vi "CreateCustomScale.vi"(8 "error in (no error)":errorcluster, 11 "DAQmx-AI":refnum<class "DAQmx-AI.lvclass">) -> (0 "error out":errorcluster, 1 "Custom Scaling":bool, 2 "Custom Scale":tag, 3 "DAQmx-AI out":refnum<class "DAQmx-AI.lvclass">)   [LabVIEW 2016, in "DAQmx-AI.lvclass"]
uses:
  DAQmx-AI.lvclass
  <vilib>/DAQmx/create/scale.llb/DAQmx Create Scale (Map Ranges).vi
  <vilib>/DAQmx/create/scale.llb/DAQmx Create Scale (Linear).vi
  <vilib>/DAQmx/create/scale.llb/DAQmx Create Scale (Polynomial).vi
  <vilib>/DAQmx/create/scale.llb/DAQmx Create Scale (Table).vi
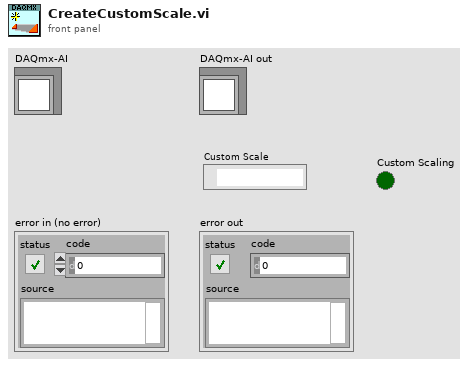
[diagram p1: front panel]
types:
  T1 = typedef "DAQmx-AI.lvclass/Scaling--Cluster.ctl" = cluster{"Scale Name":string, "Scale Type":T2, "Scaled Units":string, "Linear":T3, "Map Range":T4, "Polynomial":T5, "Table":T6}
  T2 = typedef "DAQmx-AI.lvclass/ScalingType--Enum.ctl" = enum16{"No scaling", "Linear", "Map Range", "Polynomial", "Table"}
  T3 = typedef "DAQmx-AI.lvclass/Scaling(Linear)--Cluster.ctl" = cluster{"Slope":dbl, "Intercept":dbl}
  T4 = typedef "DAQmx-AI.lvclass/Scaling(MapRange)--Cluster.ctl" = cluster{"Minimum":dbl, "Maximum":dbl}
  T5 = typedef "DAQmx-AI.lvclass/Scaling(Polynomial)--Cluster.ctl" = cluster{"forward coeff":dbl[], "reverse coeff":dbl[]}
  T6 = typedef "DAQmx-AI.lvclass/Scaling(Table)--Cluster.ctl" = cluster{"scaled values":dbl[], "pres-scaled values":dbl[]}
  T7 = typedef "DAQmx-AI.lvclass/Configuration--Cluster.ctl" = cluster{"PhysChan":tag, "Period (ms)":i64, "input terminal cfg":i32, "minimum value":dbl, "maximum value":dbl, "units":T8, "task name":string, "TDMS File Path":path, "Group Name":string}
  T8 = typedef "DAQmx-AI.lvclass/Units -- Enum.ctl" = enum16{"Volts", "Amps", "Deg F", "Deg C", "Deg R", "Kelvins", "Strain", "Ohms", "Hz", "Seconds", "Meters", "Inches", "Degrees", "Radians", "Ticks", "g", "m/s^2", "m/s", "in/s", "Pascals", "Newtons", "Pounds", "kgf", "psi", "bar", "Nm", "oz-in", "lb-in", "lb-ft", "Volts/Volt", "mVolts/Volt", "From TEDS"}
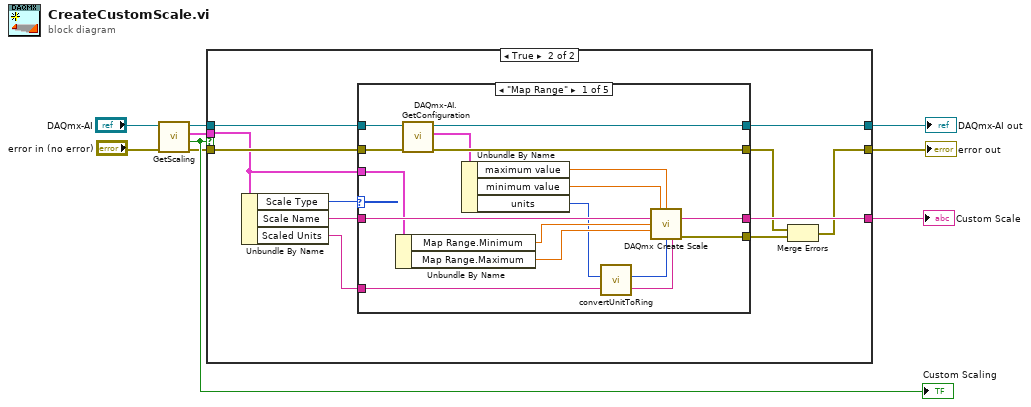
[diagram p0: block diagram]
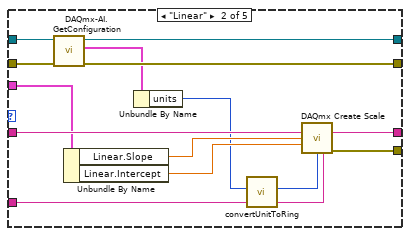
[diagram p3: hidden frame]
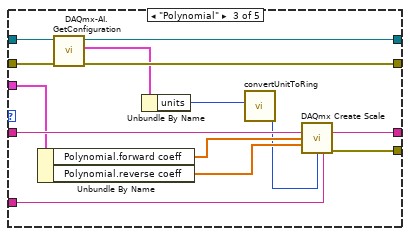
[diagram p4: hidden frame]
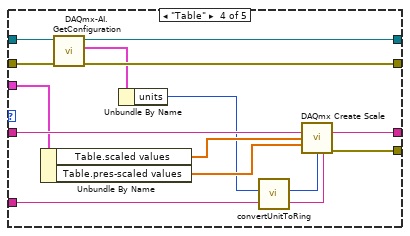
[diagram p5: hidden frame]
diagram:
  n1 = call "GetScaling.vi"("error in (no error)"="error in (no error)", "DAQmx-AI"="DAQmx-AI") -> ("error out"=w4:errorcluster, "Custom Scaling"=w7:bool, "Scaling"=w2:T1, "DAQmx-AI out"=w6:refnum<class "DAQmx-AI.lvclass">)  [unwired: 6 in]
  "Custom Scaling" <- w7
  n2 = case shown="True" w7 {
    tunnel: [w11 w19] -> w5
    tunnel: w6 -> [w11 w20]
    tunnel: w4 -> [w10 w18]
    tunnel: [w10 w13] -> w3
    tunnel: w2 -> [_ w16]
    tunnel: [_ w17] -> w1
    frame False {
    }
    frame True {
      n3 = Unbundle By Name(w16) -> ("Scale Type"=w22:T2, "Scale Name"=w21:string, "Scaled Units"=w15:string)
      n4 = case shown="\"Map Range\"" w22 {
        tunnel: w21 -> [w38 w52 w66 w80 _]
        tunnel: w20 -> [w37 w51 w65 w79 w82]
        tunnel: [w36 w50 w64 w78 w82] -> w19
        tunnel: w18 -> [w35 w49 w63 w77 w81]
        tunnel: [w34 w48 w62 w76 w81] -> w12
        tunnel: [w33 w47 w61 w75 _] -> w14
        tunnel: [w32 w46 w60 w74 _] -> w17
        tunnel: w16 -> [w26 w42 w58 w72 _]
        tunnel: w15 -> [w25 w41 w57 w71 _]
        frame "Map Range" {
          n5 = Unbundle By Name(w26) -> ("Map Range.Minimum"=w28:dbl, "Map Range.Maximum"=w27:dbl)
          n6 = call "DAQmx-AI.GetConfiguration.vi"("error in (no error)"=w35, "DAQmx-AI"=w37) -> ("error out"=w34:errorcluster, "Configuration"=w31:T7, "DAQmx-AI out"=w36:refnum<class "DAQmx-AI.lvclass">)  [unwired: 7 in]
          n7 = Unbundle By Name(w31) -> ("maximum value"=w30:dbl, "minimum value"=w29:dbl, "units"=w23:T8)
          n8 = call "convertUnitToRing.vi"("Units"=w23) -> ("DAQmx units (Ring)"=w24:i32)  [unwired: 10 in]
          n9 = call-poly <vilib>:"DAQmx Create Scale.vi"("pre-scaled minimum"=w29, "pre-scaled maximum"=w30, "name"=w38, "scaled minimum"=w28, "scaled maximum"=w27, "pre-scaled units"=w24, "scaled units"=w25) -> ("scale out"=w32:tag, "error out"=w33:errorcluster)  [unwired: 7 in]
        }
        frame "Linear" {
          n10 = call "DAQmx-AI.GetConfiguration.vi"("error in (no error)"=w49, "DAQmx-AI"=w51) -> ("error out"=w48:errorcluster, "Configuration"=w45:T7, "DAQmx-AI out"=w50:refnum<class "DAQmx-AI.lvclass">)  [unwired: 7 in]
          n11 = Unbundle By Name(w42) -> ("Linear.Slope"=w44:dbl, "Linear.Intercept"=w43:dbl)
          n12 = Unbundle By Name(w45) -> ("units"=w40:T8)
          n13 = call "convertUnitToRing.vi"("Units"=w40) -> ("DAQmx units (Ring)"=w39:i32)  [unwired: 10 in]
          n14 = call-poly <vilib>:"DAQmx Create Scale.vi"("name"=w52, "slope"=w44, "y-intercept"=w43, "pre-scaled units"=w39, "scaled units"=w41) -> ("scale out"=w46:tag, "error out"=w47:errorcluster)  [unwired: 9 in]
        }
        frame "Polynomial" {
          n15 = Unbundle By Name(w58) -> ("Polynomial.forward coeff"=w56:dbl[], "Polynomial.reverse coeff"=w55:dbl[])
          n16 = call "DAQmx-AI.GetConfiguration.vi"("error in (no error)"=w63, "DAQmx-AI"=w65) -> ("error out"=w62:errorcluster, "Configuration"=w59:T7, "DAQmx-AI out"=w64:refnum<class "DAQmx-AI.lvclass">)  [unwired: 7 in]
          n17 = Unbundle By Name(w59) -> ("units"=w54:T8)
          n18 = call "convertUnitToRing.vi"("Units"=w54) -> ("DAQmx units (Ring)"=w53:i32)  [unwired: 10 in]
          n19 = call-poly <vilib>:"DAQmx Create Scale.vi"("name"=w66, "forward coeff"=w56, "reverse coeff"=w55, "pre-scaled units"=w53, "scaled units"=w57) -> ("scale out"=w60:tag, "error out"=w61:errorcluster)  [unwired: 9 in]
        }
        frame "Table" {
          n20 = Unbundle By Name(w72) -> ("Table.scaled values"=w70:dbl[], "Table.pres-scaled values"=w69:dbl[])
          n21 = call "DAQmx-AI.GetConfiguration.vi"("error in (no error)"=w77, "DAQmx-AI"=w79) -> ("error out"=w76:errorcluster, "Configuration"=w73:T7, "DAQmx-AI out"=w78:refnum<class "DAQmx-AI.lvclass">)  [unwired: 7 in]
          n22 = Unbundle By Name(w73) -> ("units"=w68:T8)
          n23 = call "convertUnitToRing.vi"("Units"=w68) -> ("DAQmx units (Ring)"=w67:i32)  [unwired: 10 in]
          n24 = call-poly <vilib>:"DAQmx Create Scale.vi"("name"=w80, "scaled values"=w70, "pre-scaled values"=w69, "pre-scaled units"=w67, "scaled units"=w71) -> ("scale out"=w74:tag, "error out"=w75:errorcluster)  [unwired: 9 in]
        }
        frame "No scaling" {
        }
      }
      n25 = Merge Errors(w12, w14) -> (w13:errorcluster)
    }
  }
  "Custom Scale" <- w1
  "error out" <- w3
  "DAQmx-AI out" <- w5
